vi "GetProperties.vi"(8 "error in":errorcluster, 11 "Page in":refnum<class "Page.lvclass">) -> (0 "error out":errorcluster, 3 "Page out":refnum<class "Page.lvclass">)   [LabVIEW 2014, in "Page.lvclass"]
uses:
  Page.lvclass
  Page.lvclass/Page.ctl
  Generic/Generic.lvclass
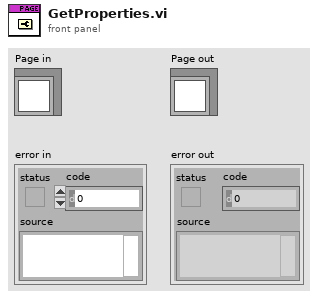
[diagram p1: front panel]
types:
  T1 = typedef "LVForegroundBackgroundColorsTypeDef.ctl" = cluster{"FG Color":u32, "BG Color":u32}
  T2 = enum32{"Page Enabled", "Page Disabled", "Page Disabled & Grayed"}
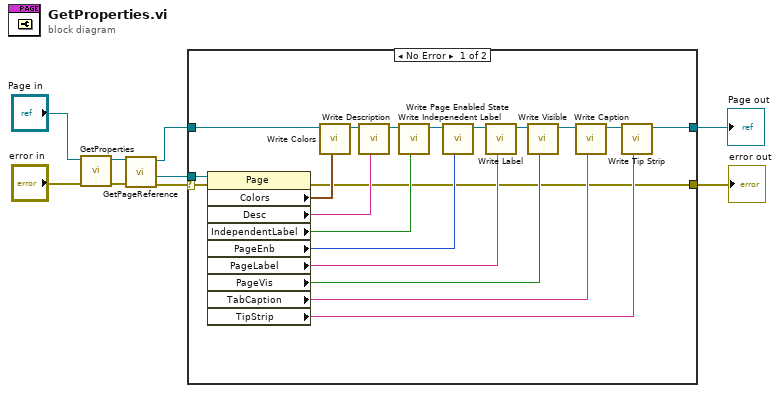
[diagram p0: block diagram]
diagram:
  n1 = call-parent "GetProperties.vi"("error in"="error in", "Generic in"="Page in") -> ("error out"=w6:errorcluster, "Generic out"=w7:refnum<class "Page.lvclass">)  [unwired: 8 in]
  n2 = call "GetPageReference.vi"("error in"=w6, "Page in"=w7) -> ("error out"=w5:errorcluster, "page reference"=w4:refnum<vi>, "Page out"=w2:refnum<class "Page.lvclass">)  [unwired: 7 in]
  n3 = case shown="No Error" w5 {
    selector: w5 -> [w29 w30]
    tunnel: w4 -> [w28 _]
    tunnel: [w12 w31] -> w3
    tunnel: w2 -> [w11 w31]
    tunnel: [w10 w30] -> w1
    frame No Error {
      n4 = property class="Page"(reference=w28, error in=w29) -> (error out=w10:errorcluster, "Colors"=w27:T1, "Desc"=w25:string, "IndependentLabel"=w23:bool, "PageEnb"=w21:T2, "PageLabel"=w16:string, "PageVis"=w15:bool, "TabCaption"=w14:string, "TipStrip"=w13:string)  [unwired: 1 out]
      n5 = call "Write Colors.vi"("Colors"=w27, "Page in"=w11) -> ("Page out"=w26:refnum<class "Page.lvclass">)  [unwired: 7 in]
      n6 = call "Write Description.vi"("Description"=w25, "Page in"=w26) -> ("Page out"=w24:refnum<class "Page.lvclass">)  [unwired: 7 in]
      n7 = call "Write Indepenedent Label.vi"("Indepenedent Label"=w23, "Page in"=w24) -> ("Page out"=w22:refnum<class "Page.lvclass">)  [unwired: 7 in]
      n8 = call "Write Page Enabled State.vi"("Page Enabled State"=w21, "Page in"=w22) -> ("Page out"=w20:refnum<class "Page.lvclass">)  [unwired: 7 in]
      n9 = call "Write Label.vi"("Label"=w16, "Page in"=w20) -> ("Page out"=w19:refnum<class "Page.lvclass">)  [unwired: 7 in]
      n10 = call "Write Visible.vi"("Visible"=w15, "Page in"=w19) -> ("Page out"=w18:refnum<class "Page.lvclass">)  [unwired: 7 in]
      n11 = call "Write Caption.vi"("Caption"=w14, "Page in"=w18) -> ("Page out"=w17:refnum<class "Page.lvclass">)  [unwired: 7 in]
      n12 = call "Write Tip Strip.vi"("Tip Strip"=w13, "Page in"=w17) -> ("Page out"=w12:refnum<class "Page.lvclass">)  [unwired: 7 in]
    }
    frame Error {
    }
  }
  "error out" <- w1
  "Page out" <- w3
